vi "Close Async VIs.vi"(6 "TopLevel VI":refnum<vi>, 8 "error in (no error)":errorcluster, 10 "Error Handling Refs":T1, 11 "Async VI":refnum<vi>[](array[refnum])) -> (0 "error out":errorcluster)   [LabVIEW 2015, in "Waveform-Processing-Custom-Device Engine.lvlib" / "Inline Async API.lvlib"]
uses:
  Inline Async API.lvlib
  Error Handling API/Controls/Error Handling Cluster.ctl
  Error Handling API/Print/Display and Log Custom Device Error.vi
  <vilib>/NI Veristand/Custom Device Tools/Custom Device Utility Library/NI VeriStand - Print Debug String.vi
  Error Handling API/Error Handling API.lvlib
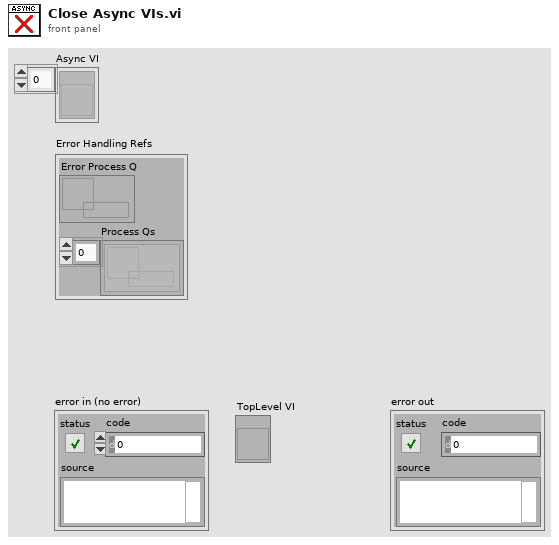
[diagram p1: front panel]
types:
  T1 = typedef "Waveform-Processing-Custom-Device Engine.lvlib/Error Handling API.lvlib/Error Handling Cluster.ctl" = cluster{"Error Process Q":refnum<queue>, "Process Qs":refnum<queue>[]}
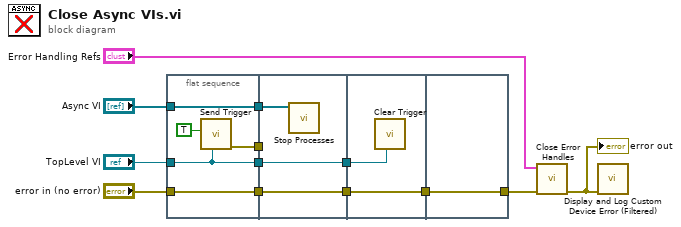
[diagram p0: block diagram]
diagram:
  n1 = flat-sequence {
    tunnel: [w17] -> w13
    tunnel: "TopLevel VI" -> [w16]
    tunnel: [w16] -> w12
    tunnel: "Async VI" -> [w15]
    tunnel: [w15] -> w11
    tunnel: [w14] -> w10
    tunnel: "error in (no error)" -> [w14]
    tunnel: w13 -> [_]
    tunnel: w12 -> [w21]
    tunnel: [w21] -> w9
    tunnel: w11 -> [w20]
    tunnel: [w19] -> w8
    tunnel: w10 -> [w19]
    tunnel: w9 -> [w23]
    tunnel: w8 -> [w22]
    tunnel: [w22] -> w7
    tunnel: [w24] -> w4
    tunnel: w7 -> [w24]
    frame #0 {
      n2 = call "Send Trigger.vi"("Parent VI"=w16, "notification"=TRUE) -> ("error out"=w17:errorcluster)  [unwired: 9 in]
    }
    frame #1 {
      n3 = call "Stop Processes.vi"("VI Refs"=w20) -> ()  [unwired: 11 in]
    }
    frame #2 {
      n4 = call "Clear Trigger.vi"("Parent VI"=w23) -> ()  [unwired: 10 in, 1 out]
    }
    frame #3 {
    }
  }
  n5 = call "Close Error Handles.vi"("error in"=w4, "Error Handling Cluster"="Error Handling Refs") -> ("error out"=w6:errorcluster)  [unwired: 9 in]
  "error out" <- w6
  n6 = call "Display and Log Custom Device Error (Filtered).vi"("error in (no error)"=w6) -> ()  [unwired: 11 in]
